vi "getfreqandpwr.vi"(11 "VISA resource name":refnum<visa-resource-name>) -> (0 "Freq":dbl format="%.7f", 3 "RF Detector Pwr dBm":dbl=-67.9609375 format="%_5g", 4 "error?":bool, 8 "EOS":bool)   [LabVIEW 2012]
uses:
  <vilib>/Utility/error.llb/DialogType.ctl
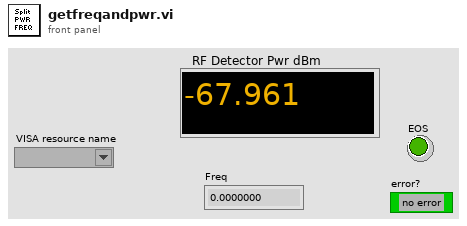
[diagram p1: front panel]
types:
  T1 = typedef "DialogType.ctl" = u16
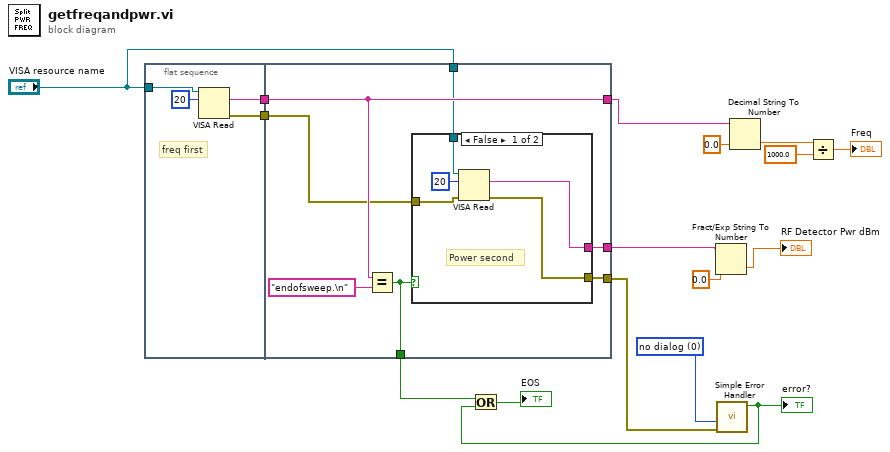
[diagram p0: block diagram]
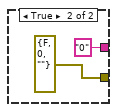
[diagram p2: hidden frame]
diagram:
  w4 = T1 0 items=["no dialog", "OK message", "continue or stop message", "OK message + warnings", "continue/stop + warnings"] ("type of dialog (OK msg:1)")
  n1 = flat-sequence {
    tunnel: "VISA resource name" -> [w19]
    tunnel: [w18] -> w12
    tunnel: [w17] -> w6
    tunnel: [w24] -> w11
    tunnel: w12 -> [w24]
    tunnel: [w26] -> w3
    tunnel: [w25] -> w9
    tunnel: "VISA resource name" -> [w23]
    tunnel: w6 -> [w22]
    tunnel: [w21] -> w5
    frame #0 {
      # "freq first"
      n2 = VISA Read(VISA resource name=w19, byte count=u32 20) -> (read buffer=w18:string, error out=w17:errorcluster)  [unwired: 1 in, 2 out]
    }
    frame #1 {
      n3 = Equal?(x=w24, y="endofsweep.\n") -> (x = y?=w26:bool)
      n4 = case shown="False" w26 {
        tunnel: [w31 "0" ("read buffer")] -> w25
        tunnel: w23 -> [w30 _]
        tunnel: w22 -> [w29 _]
        tunnel: [w28 errorcluster {"status"=FALSE, "code"=0, "source"=""} ("error out")] -> w21
        frame False {
          # "Power second"
          n5 = VISA Read(VISA resource name=w30, byte count=u32 20, error in (no error)=w29) -> (read buffer=w31:string, error out=w28:errorcluster)  [unwired: 2 out]
        }
        frame True {
        }
      }
    }
  }
  n6 = Fract/Exp String To Number(string=w9, default (0 dbl)=0.0 ("default (0 I32)")) -> (number=→"RF Detector Pwr dBm":dbl)  [unwired: 2 in, 1 out]
  n7 = call <vilib>:"Simple Error Handler.vi"("type of dialog (OK msg:1)"=w4, "error in (no error)"=w5) -> ("error?"=w1:bool)  [unwired: 7 out]
  "error?" <- w1
  n8 = Or(x=w3, y=w1) -> (x .or. y?=→"EOS":bool)
  n9 = Decimal String To Number(string=w11, default (0L)=0.0 ("default (0 I32)")) -> (number=w16:dbl)  [unwired: 1 in, 1 out]
  n10 = Divide(x=w16, y=1000.0) -> (x/y=→"Freq":dbl)
